vi "Destroy.vi"(8 "error in (no error)":errorcluster, 10 "Retrieve Commands? (F)":bool, 11 "queue in":refnum<queue>) -> (0 "error out":errorcluster, 2 "Command":T1[](array[typedef]), 3 "queue name":string)   [LabVIEW 2013, in "命令队列.lvlib"]
uses:
  <vilib>/CommandQueue/Command.ctl
  Command.ctl
  <vilib>/CommandQueue/Command Queue.lvlib
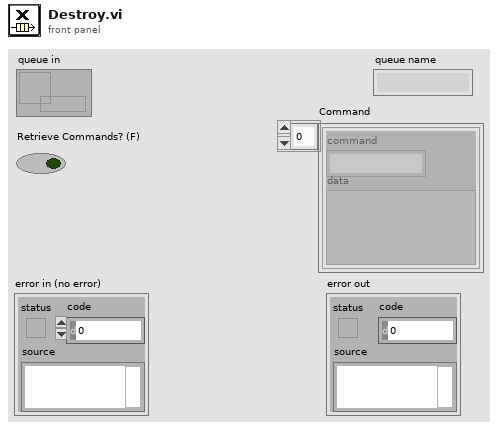
[diagram p1: front panel]
types:
  T1 = typedef "Command Queue.lvlib/Command.ctl" = cluster{"command":string, "data":variant}
  T2 = typedef "命令队列.lvlib/Command.ctl" = cluster{"command":string, "data":variant}
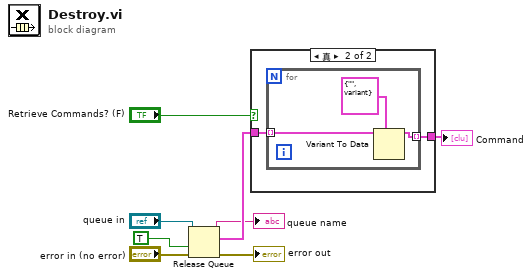
[diagram p0: block diagram]
diagram:
  n1 = Release Queue(queue="queue in", force destroy? (F)=TRUE, error in (no error)="error in (no error)") -> (queue name=→"queue name":string, remaining elements=w5:cluster{"command":string, "data":variant}[], error out=→"error out":errorcluster)
  n2 = case shown="真" "Retrieve Commands? (F)" {
    tunnel: w5 -> [_ w10]
    tunnel: [_ w9] -> w6
    frame False {
    }
    frame True {
      n3 = for {
        tunnel: w10 -> [w13] mode=indexing
        tunnel: [w12] -> w9 mode=indexing
        n4 = Variant To Data(type=T2 {"command"="", "data"=variant} ("command queue element"), Variant=w13) -> (data=w12:T2)  [unwired: 1 in, 1 out]
      }
    }
  }
  "Command" <- w6
